vi "set_params.vi"(8 "error in (no error)":errorcluster caption="entrée d'erreur (pas d'erreur)", 11 "LassoLarsIC.lvclass 2":refnum<class "LassoLarsIC.lvclass">) -> (0 "error out":errorcluster caption="sortie d'erreur", 3 "LassoLarsIC.lvclass":refnum<class "LassoLarsIC.lvclass">)   [LabVIEW 2020, in "LassoLarsIC.lvclass"]
uses:
  LassoLarsIC.lvclass
  LassoLarsIC.lvclass/LassoLarsIC.ctl
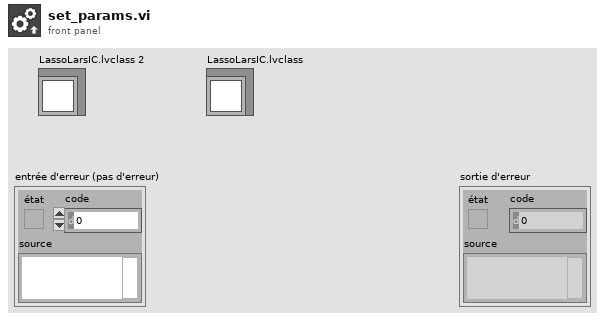
[diagram p1: front panel]
types:
  T1 = typedef "lasso_lars_ic_params.ctl" = cluster{"criterion":string, "fit_intercept":bool, "verbose":cluster{"verbose_type":string, "verbose_bool":bool, "verbose_int":dbl}, "normalize":bool, "precompute":cluster{"precompute_type":string, "precompute_bool":bool, "precompute_list":dbl[][]}, "max_iter":dbl, "copy_X":bool, "positive":bool}
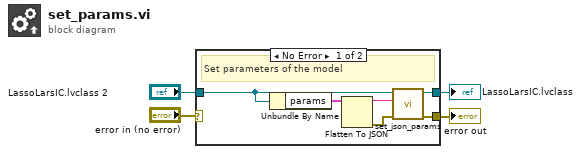
[diagram p0: block diagram]
diagram:
  n1 = case shown="No Error" "error in (no error)" {
    selector: "error in (no error)" -> [_ w12]
    tunnel: [w7 w12] -> w3
    tunnel: [w8 w11] -> w1
    tunnel: "LassoLarsIC.lvclass 2" -> [w5 w11]
    frame No Error {
      # "Set parameters of the model"
      n2 = Unbundle By Name(w5) -> ("params"=w10:T1)
      n3 = Flatten To JSON(anything=w10) -> (JSON string=w9:string, 11:w6:errorcluster)  [unwired: 2 in]
      n4 = call-dynamic "set_json_params.vi"("error in (no error)"=w6, "params"=w9, "Model en entrée"=w5) -> ("error out"=w7:errorcluster, "Model en sortie"=w8:refnum<class "LassoLarsIC.lvclass">)  [unwired: 7 in]
    }
    frame Error {
    }
  }
  "error out" <- w3
  "LassoLarsIC.lvclass" <- w1
